vi "ADI_IMU_ADIS16470_Loop.vi"(8 "error in":errorcluster, 11 "ADI IMU DevRef":T1) -> (1 "Device Found":bool)   [LabVIEW 2017, in "ADIS16470_IMU.lvlib"]
doc: "Periodically reads the ADI MXP IMU valuse and makes data available for use elsewhere in your robot project. Place this block within PeriodicTasks.vi outside any loops."
uses:
  ADIS16470_IMU.lvlib
  ADI_IMU_ADIS16470_IMUDevRef.ctl
  <vilib>/Rock Robotics/SystemInterfaces/spilib/spi_bus.ctl
panel:
  in  "Main Name":string
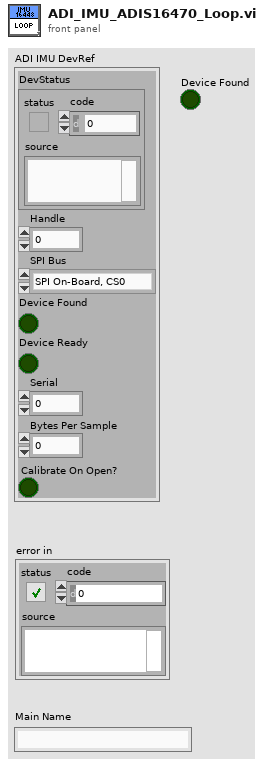
[diagram p1: front panel]
types:
  T1 = typedef "ADIS16470_IMU.lvlib/ADI_IMU_ADIS16470_IMUDevRef.ctl" = cluster{"DevStatus":errorcluster, "Handle":i32, "SPI Bus":T2, "Device Found":bool, "Device Ready":bool, "Serial":u16, "Bytes Per Sample":u16, "Calibrate On Open?":bool}
  T2 = typedef "spi_bus.ctl" = enum16{"SPI On-Board, CS0", "SPI On-Board, CS1", "SPI On-Board, CS2", "SPI On-Board, CS3", "SPI MXP", "Invalid"}
  T3 = cluster{"X Angle":dbl, "Y Angle":dbl, "Z Angle":dbl}
  T4 = enum32{"Bad", "Idle", "Run top level", "Running"}
  T5 = cluster{"X Gyro":dbl, "Y Gyro":dbl, "Z Gyro":dbl, "X Accel":dbl, "Y Accel":dbl, "Z Accel":dbl, "Temp":dbl}
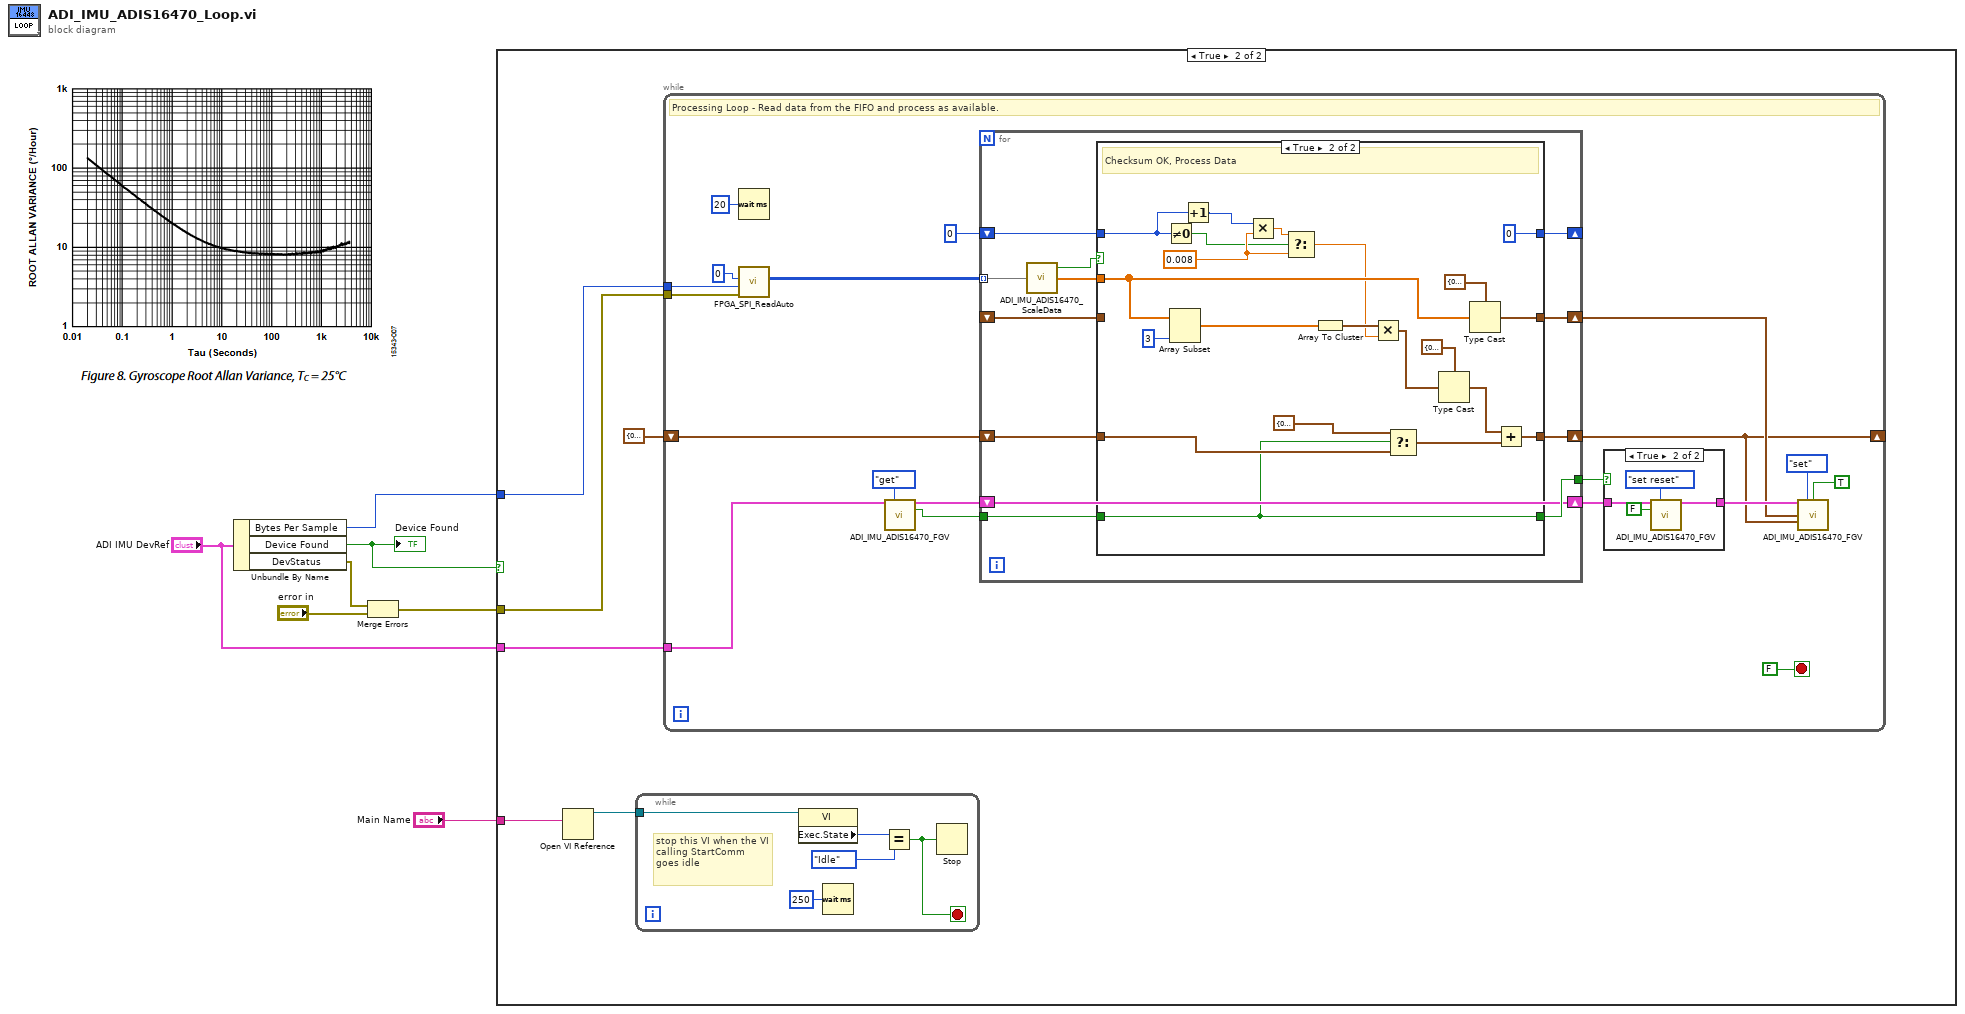
[diagram p0: block diagram]
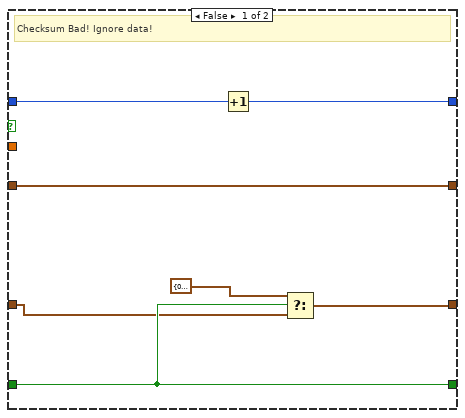
[diagram p3: hidden frame]
diagram:
  n1 = Unbundle By Name("ADI IMU DevRef") -> ("Bytes Per Sample"=w2:u16, "Device Found"=w4:bool, "DevStatus"=w5:errorcluster)
  "Device Found" <- w4
  n2 = Merge Errors(w5, "error in") -> (w1:errorcluster)
  n3 = case shown="True" w4 {
    tunnel: "Main Name" -> [_ w12]
    tunnel: "ADI IMU DevRef" -> [_ w8]
    tunnel: w2 -> [_ w11]
    tunnel: w1 -> [_ w10]
    frame False {
    }
    frame True {
      n4 = Open VI Reference(vi path=w12) -> (vi reference=w13:refnum<vi>)  [unwired: 1 in, 5 out]
      n5 = while {
        tunnel: w13 -> [w15]
        stop <- w14 stop-if-true
        # "stop this VI when the VI calling StartComm goes idle"
        n6 = property class="VI"(reference=w15) -> ("Exec.State"=w17:T4)  [unwired: 1 in, 2 out]
        n7 = Wait (ms)(milliseconds to wait=u32 250) -> ()  [unwired: 1 out]
        n8 = Equal?(x=w17, y=T4."Idle" ("Execution:State")) -> (x = y?=w14:bool)
        n9 = Stop(stop? (T)=w14) -> ()
      }
      n10 = while {
        tunnel: w8 -> [w23]
        tunnel: w11 -> [w30]
        tunnel: w10 -> [w29]
        shift-right: [w21] -> _
        shift-left: T3 {"X Angle"=0.0, "Y Angle"=0.0, "Z Angle"=0.0} ("IMU Angles") -> [w27]
        stop <- FALSE stop-if-true
        # "Processing Loop - Read data from the FIFO and process as available."
        n11 = Wait (ms)(milliseconds to wait=u32 20) -> ()  [unwired: 1 out]
        n12 = call <vilib>:"FPGA_SPI_ReadAuto.vi"("error in (no error)"=w29, "Bytes per Sample"=w30, "Samples to Read"=u32 0) -> ("Data"=w26:u8[][])  [unwired: 7 in, 1 out]
        n13 = call "ADI_IMU_ADIS16470_FGV.vi"("ADI IMU DevRef"=w23, "Operation"=enum16{"set", "get", "set reset"}."get") -> ("ADI IMU DevRef Out"=w24:T1, "Reset Out"=w22:bool)  [unwired: 8 in, 4 out]
        n14 = for {
          tunnel: [w42] -> w32
          shift-right: [w48] -> w21
          shift-left: w27 -> [w49]
          shift-right: [w38] -> w34
          shift-left: w24 -> [w38]
          tunnel: w26 -> [w45] mode=indexing
          tunnel: w22 -> [w43]
          shift-right: [w40] -> _
          shift-left: 0 -> [w41]
          shift-right: [w46] -> w28
          shift-left: _ -> [w39]
          n15 = call "ADI_IMU_ADIS16470_ScaleData.vi"("Received Data"=w45) -> ("Data Array"=w47:dbl[], "Data Good?"=w44:bool)  [unwired: 3 in]
          n16 = case shown="True" w44 {
            tunnel: w49 -> [w51 w77]
            tunnel: [w50 w76] -> w48
            tunnel: w47 -> [_ w66]
            tunnel: [w54 w65] -> w46
            tunnel: [w52 w64] -> w42
            tunnel: w43 -> [w52 w64]
            tunnel: w41 -> [w56 w57]
            tunnel: [w55 0] -> w40
            tunnel: w39 -> [w54 _]
            frame False {
              # "Checksum Bad! Ignore data!"
              n17 = Increment(x=w56) -> (x+1=w55:i32)
              n18 = Select(t=T3 {"X Angle"=0.0, "Y Angle"=0.0, "Z Angle"=0.0} ("IMU Angles"), s=w52, f=w51) -> (s? t:f=w50:T3)
            }
            frame True {
              w61 = 0.008
              # "Checksum OK, Process Data"
              n19 = Not Equal To 0?(x=w57) -> (x != 0?=w60:bool)
              n20 = Array Subset(array=w66, length=3) -> (w74:dbl[])  [unwired: 1 in]
              n21 = Increment(x=w57) -> (x+1=w58:i32)
              n22 = Multiply(x=w58, y=w61) -> (x*y=w62:dbl)
              n23 = Select(t=w62, s=w60, f=w61) -> (s? t:f=w63:dbl)
              n24 = Array To Cluster(array=w74) -> (cluster=w73:cluster{"[0]":dbl, "[1]":dbl, "[2]":dbl})
              n25 = Multiply(x=w73, y=w63) -> (x*y=w69:cluster{"[0]":dbl, "[1]":dbl, "[2]":dbl})
              n26 = Select(t=T3 {"X Angle"=0.0, "Y Angle"=0.0, "Z Angle"=0.0} ("IMU Angles"), s=w64, f=w77) -> (s? t:f=w72:T3)
              n27 = Type Cast(type=T3 {"X Angle"=0.0, "Y Angle"=0.0, "Z Angle"=0.0} ("IMU Angles"), x=w69) -> (*(type *) &x=w70:T3)
              n28 = Type Cast(type=T5 {"X Gyro"=0.0, "Y Gyro"=0.0, "Z Gyro"=0.0, "X Accel"=0.0, "Y Accel"=0.0, "Z Accel"=0.0, "Temp"=0.0} ("IMU Data"), x=w66) -> (*(type *) &x=w65:T5)
              n29 = Add(x=w70, y=w72) -> (x+y=w76:T3)
            }
          }
        }
        n30 = case shown="True" w32 {
          tunnel: [w78 w81] -> w35
          tunnel: w34 -> [w78 w80]
          frame False {
          }
          frame True {
            n31 = call "ADI_IMU_ADIS16470_FGV.vi"("ADI IMU DevRef"=w80, "Operation"=enum16{"set", "get", "set reset"}."set reset", "Reset"=FALSE) -> ("ADI IMU DevRef Out"=w81:T1)  [unwired: 7 in, 5 out]
          }
        }
        n32 = call "ADI_IMU_ADIS16470_FGV.vi"("ADI IMU DevRef"=w35, "Operation"=enum16{"set", "get", "set reset"}."set", "Sensor Ready?"=TRUE, "IMU Data"=w28, "IMU Angles"=w21) -> ()  [unwired: 5 in, 6 out]
      }
    }
  }
